vi "NavX_Main.vi"   [LabVIEW 2017]
uses:
  <vilib>/Rock Robotics/WPI/ThirdParty/Sensors/navX/_TypeDefs/FRIC_navX_DeviceNumbersTypeDef.ctl
  <vilib>/Rock Robotics/WPI/ThirdParty/Sensors/navX/_Processing Loop/FRIC_navX_Internal_Serial_ProcessingLoop.vi
types:
  T1 = typedef "FRIC_navX_DeviceNumbersTypeDef.ctl" = enum16{"Dev0", "Dev1", "Dev2", "Dev3"}
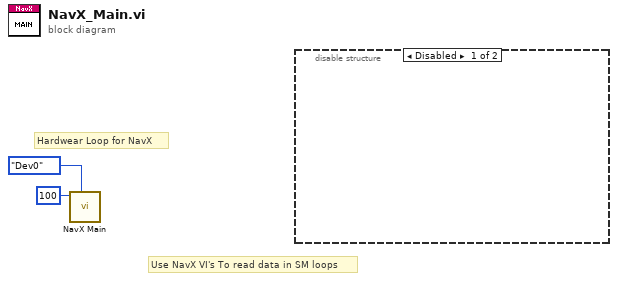
[diagram p0: block diagram]
diagram:
  # "Use NavX VI's To read data in SM loops"
  # "Hardwear Loop for NavX"
  n1 = call-poly <vilib>:"NavX Main.vi"("Device Number"=FRIC_navX_DeviceNumbersTypeDef."Dev0", "Rate (4Hz-200Hz)"=u8 100) -> ()  [unwired: 10 in]
  n2 = disable-structure shown="Disabled" {
    frame Disabled {
    }
    frame Enabled {
    }
  }
